vi "Set Custom Route Properties.vi"(8 "error in (no error)":errorcluster, 10 "Routes":T1, 11 "Item Ref in":T3 format="%.0x") -> (0 "error out":errorcluster, 3 "Item Ref out":T3 format="%.0x")   [LabVIEW 2011, in "Chassis TimeSync System Explorer.lvlib"]
uses:
  Chassis TimeSync System Explorer.lvlib
  <vilib>/NI Veristand/Custom Device API/Custom Device Item Ref.ctl
  Shared/Routes.ctl
  Shared/Route.ctl
  Shared/Constants.vi
  <vilib>/NI Veristand/Custom Device API/Set Item Property (String).vi
  Shared/Chassis TimeSync Shared.lvlib
  <vilib>/NI Veristand/Custom Device API/Custom Device API.lvlib
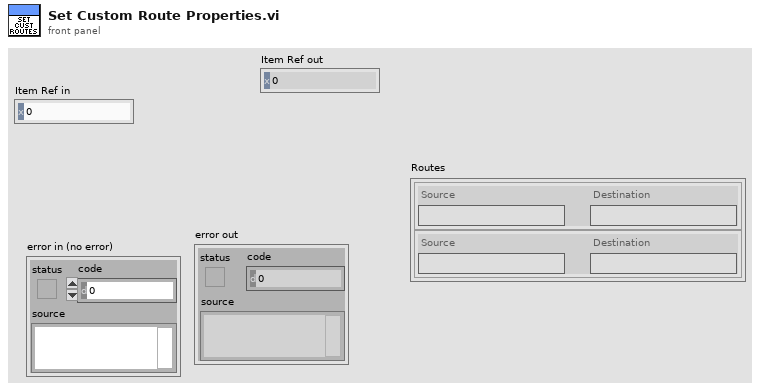
[diagram p1: front panel]
types:
  T1 = typedef "Chassis TimeSync Shared.lvlib/Routes.ctl" = T2[]
  T2 = typedef "Chassis TimeSync Shared.lvlib/Route.ctl" = cluster{"Source":string, "Destination":string}
  T3 = typedef "Custom Device API.lvlib/Custom Device Item Ref.ctl" = u64
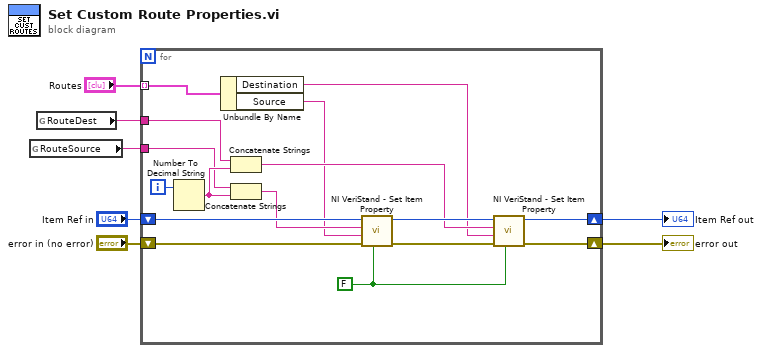
[diagram p0: block diagram]
diagram:
  n1 = global read "Constants.vi" "RouteSource"() -> (w5:string)
  n2 = global read "Constants.vi" "RouteDest"() -> (w4:string)
  n3 = for {
    shift-right: [w13] -> w2
    shift-left: "error in (no error)" -> [w23]
    tunnel: w5 -> [w16]
    tunnel: w4 -> [w15]
    tunnel: "Routes" -> [w11] mode=indexing
    shift-right: [w12] -> w3
    shift-left: "Item Ref in" -> [w22]
    i -> [w21]
    w8 = FALSE ("Binary String (T)")
    n4 = Number To Decimal String(number=w21) -> (decimal integer string=w17:string)  [unwired: 1 in]
    n5 = Unbundle By Name(w11) -> ("Destination"=w9:string, "Source"=w10:string)
    n6 = Concatenate Strings(w15, w17) -> (w14:string)
    n7 = Concatenate Strings(w16, w17) -> (w20:string)
    n8 = call-poly <vilib>:"NI VeriStand - Set Item Property.vi"("Binary String (T)"=w8, "error in (no error)"=w23, "Value"=w10, "Property Name"=w20, "Item Ref in"=w22) -> ("error out"=w19:errorcluster, "Item Ref out"=w18:T3)  [unwired: 4 in, 1 out]
    n9 = call-poly <vilib>:"NI VeriStand - Set Item Property.vi"("Binary String (T)"=w8, "error in (no error)"=w19, "Value"=w9, "Property Name"=w14, "Item Ref in"=w18) -> ("error out"=w13:errorcluster, "Item Ref out"=w12:T3)  [unwired: 4 in, 1 out]
  }
  "error out" <- w2
  "Item Ref out" <- w3
